vi "testDTR.vi"(3 "error in":errorcluster, 4 "File Path":path[](array[path]), 5 "Dry Test Run":bool) -> (0 "error out":errorcluster, 1 "Solenoid Outputs":bool[](array[boolean]), 2 "DTR Done":bool)   [LabVIEW 2021]
uses:
  <vilib>/Utility/file.llb/Read Delimited Spreadsheet (string).vi
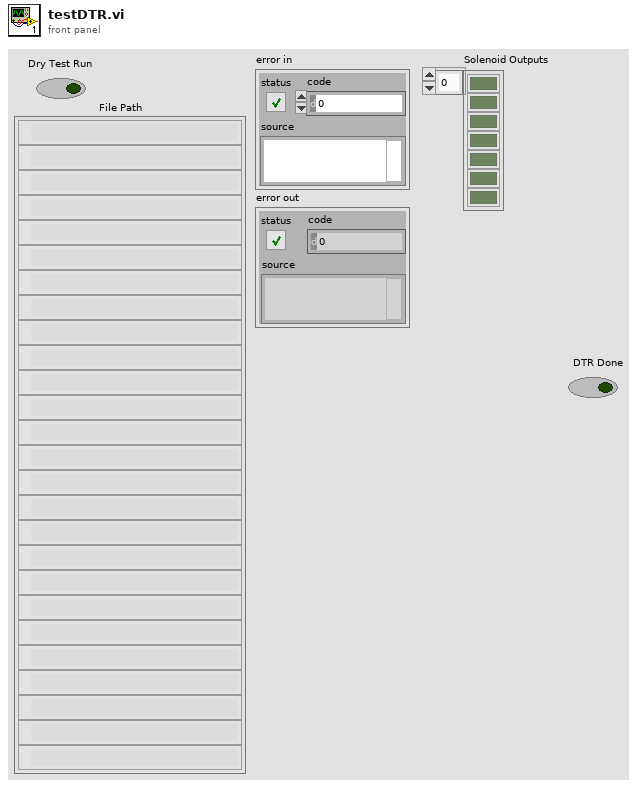
[diagram p1: front panel]
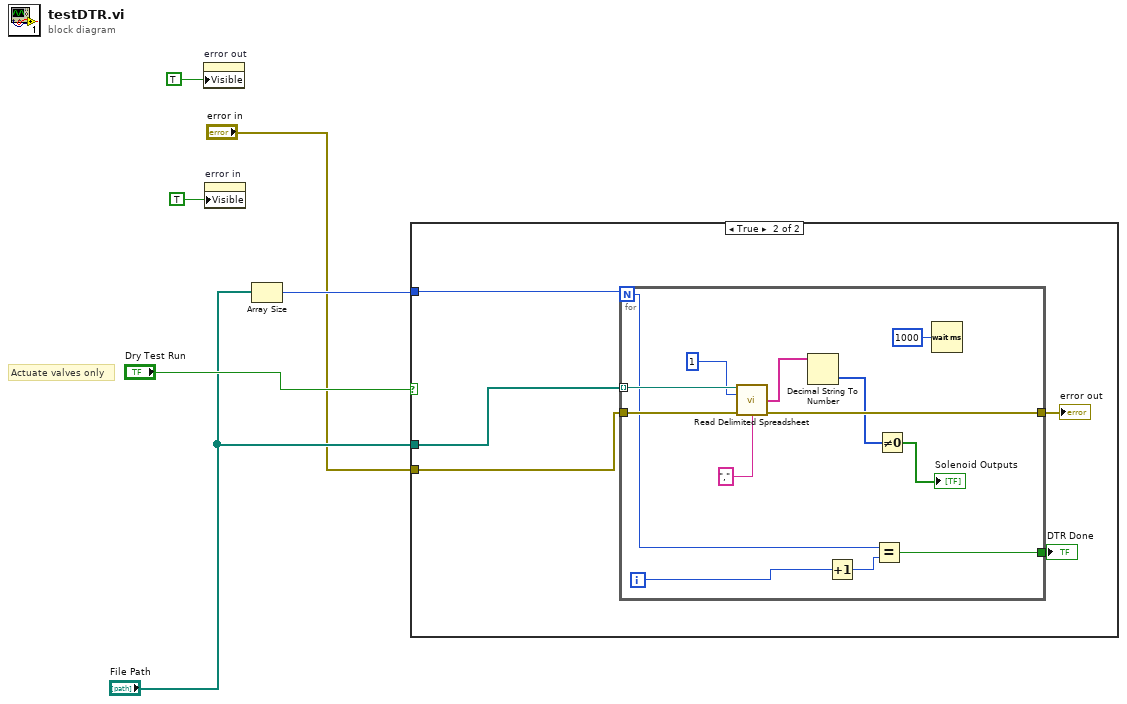
[diagram p0: block diagram]
diagram:
  # "Actuate valves only"
  n1 = property on="error out" class="Clust (strict)"("Visible"=TRUE) -> ()  [unwired: 2 in, 2 out]
  n2 = property on="error in" class="Clust (strict)"("Visible"=TRUE) -> ()  [unwired: 2 in, 2 out]
  n3 = Array Size(array="File Path") -> (size(s)=w3:i32)
  n4 = case shown="True" "Dry Test Run" {
    tunnel: w3 -> [_ w7]
    tunnel: "File Path" -> [_ w8]
    tunnel: "error in" -> [_ w9]
    frame False {
    }
    frame True {
      n5 = for {
        N: w7 -> [w15]
        tunnel: w8 -> [w24] mode=indexing
        tunnel: w9 -> [w21]
        tunnel: [w20] -> w10
        tunnel: [w14] -> w11
        i -> [w16]
        n6 = call-poly <vilib>:"Read Delimited Spreadsheet.vi"("file path (dialog if empty)"=w24, "number of rows (all:-1)"=1, "error in (no error)"=w21, "delimiter (\\t)"="," ("delimiter (\\t)")) -> ("first row"=w19:string[], "error out"=w20:errorcluster)  [unwired: 6 in, 4 out]
        n7 = Decimal String To Number(string=w19) -> (number=w18:i32[])  [unwired: 2 in, 1 out]
        n8 = Increment(x=w16) -> (x+1=w17:i32)
        n9 = Equal?(x=w15, y=w17) -> (x = y?=w14:bool)
        n10 = Not Equal To 0?(x=w18) -> (x != 0?=→"Solenoid Outputs":bool[])
        n11 = Wait (ms)(milliseconds to wait=u32 1000) -> ()  [unwired: 1 out]
      }
      "error out" <- w10
      "DTR Done" <- w11
    }
  }
